vi "Update Chart Buffer Data--SubVI.vi"(9 "Chart Data":dbl[](array[numeric]), 10 "Chart Buffer In":dbl[][](array[numeric]), 11 "Chart Index In":i32) -> (2 "Chart Buffer Out":dbl[][](array[numeric]), 3 "Chart Index Out":i32)   [LabVIEW 2025, in "Chart.lvlib"]
doc: "<b>Note:</b> This VI was modified by the <b>Validate DQMH Module</b> tool to turn off automatic error handling."
uses:
  Chart.lvlib
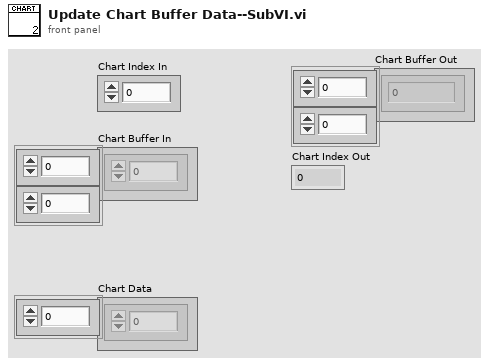
[diagram p1: front panel]
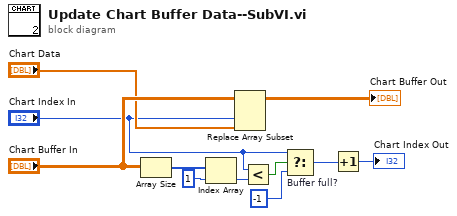
[diagram p0: block diagram]
diagram:
  n1 = Array Size(array="Chart Buffer In") -> (size(s)=w10:i32[])
  n2 = Index Array(array=w10, index=1) -> (element=w8:i32)
  n3 = Replace Array Subset(array="Chart Buffer In", new element="Chart Data", index (col)="Chart Index In") -> (→"Chart Buffer Out":dbl[][])  [unwired: 1 in]
  n4 = Less?(x="Chart Index In", y=w8) -> (x < y?=w11:bool)
  n5 = Select "Buffer full?"(t="Chart Index In", s=w11, f=-1) -> (s? t:f=w7:i32)
  n6 = Increment(x=w7) -> (x+1=→"Chart Index Out":i32)
